vi "write_txt_isotope_value1_vaue_2.vi"(8 "error in (no error)":errorcluster, 11 "DataLoggingText in":refnum<class "DataLogging.lvclass">) -> (0 "error out":errorcluster, 3 "DataLoggingText out":refnum<class "DataLogging.lvclass">)   [LabVIEW 2018, in "DataLogging.lvclass"]
doc: "writes data into a text file.\ndata are:\n- isotope name\n- value 1\n- value 2"
uses:
  DataLogging.lvclass
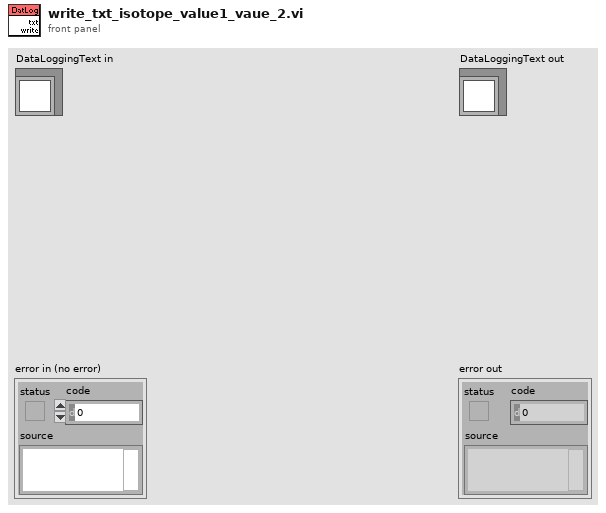
[diagram p1: front panel]
types:
  T1 = typedef "ValueArray.ctl" = string[]
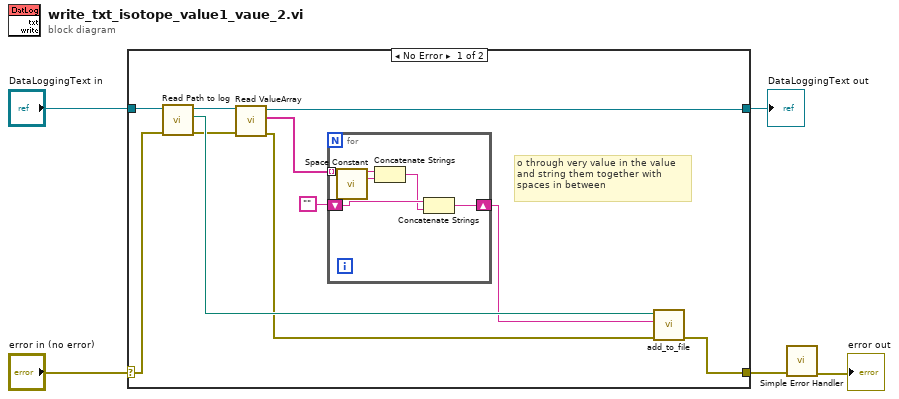
[diagram p0: block diagram]
diagram:
  n1 = case shown="No Error" "error in (no error)" {
    selector: "error in (no error)" -> [w13 w23]
    tunnel: [w14 w23] -> w2
    tunnel: [w10 w22] -> w3
    tunnel: "DataLoggingText in" -> [w16 w22]
    frame No Error {
      # "o through very value in the value\nand string them together with \nspaces in between"
      n2 = call-dynamic "Read Path to log.vi"("error in (no error)"=w13, "DataLoggingText in"=w16) -> ("error out"=w11:errorcluster, "Path to log"=w15:path, "DataLoggingText out"=w12:refnum<class "DataLogging.lvclass">)  [unwired: 7 in]
      n3 = call-dynamic "Read ValueArray.vi"("error in (no error)"=w11, "DataLogging in"=w12) -> ("error out"=w9:errorcluster, "ValueArray"=w8:T1, "DataLogging out"=w10:refnum<class "DataLogging.lvclass">)  [unwired: 7 in]
      n4 = for {
        tunnel: w8 -> [w19] mode=indexing
        shift-right: [w21] -> w7
        shift-left: "" -> [w20]
        n5 = call <vilib>:"Space Constant.vi"() -> ("String"=w18:string)
        n6 = Concatenate Strings(w19, w18) -> (w17:string)
        n7 = Concatenate Strings(w20, w17) -> (w21:string)
      }
      n8 = call "add_to_file.vi"("error in (no error)"=w9, "String"=w7, "Path to log"=w15) -> ("error out"=w14:errorcluster)  [unwired: 8 in]
    }
    frame Error {
    }
  }
  "DataLoggingText out" <- w3
  n9 = call <vilib>:"Simple Error Handler.vi"("error in (no error)"=w2) -> ("error out"=→"error out":errorcluster)  [unwired: 4 in, 4 out]
